vi "Инвертирование знака числа(5-разрядного).vi"(1 "A":T2) -> (0 "R":T1)   [LabVIEW 2013]
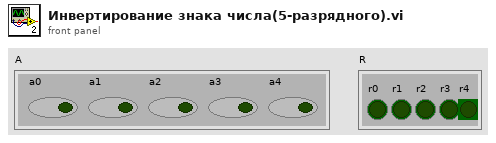
[diagram p1: front panel]
types:
  T1 = cluster{"r0":bool, "r1":bool, "r2":bool, "r3":bool, "r4":bool}
  T2 = cluster{"a0":bool, "a1":bool, "a2":bool, "a3":bool, "a4":bool}
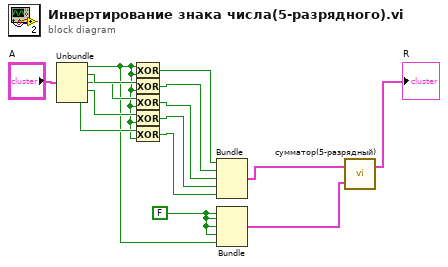
[diagram p0: block diagram]
diagram:
  w1 = FALSE
  n1 = Unbundle("A") -> ("a0"=w2:bool, "a1"=w14:bool, "a2"=w13:bool, "a3"=w12:bool, "a4"=w11:bool)
  n2 = Exclusive Or(1:w2, 2:w2) -> (0:w7:bool)
  n3 = Exclusive Or(1:w2, 2:w14) -> (0:w6:bool)
  n4 = Exclusive Or(1:w2, 2:w13) -> (0:w5:bool)
  n5 = Exclusive Or(1:w2, 2:w12) -> (0:w4:bool)
  n6 = Exclusive Or(1:w2, 2:w11) -> (0:w3:bool)
  n7 = Bundle(w7, w6, w5, w4, w3) -> (w10:cluster{bool, bool, bool, bool, bool})  [unwired: 1 in]
  n8 = Bundle(w1, w1, w1, w1, "a0"=w2) -> (w9:cluster{bool, bool, bool, bool, "a0":bool})  [unwired: 1 in]
  n9 = call "сумматор(5-разрядный).vi"("B"=w9, "A"=w10) -> ("R"=→"R":T1)  [unwired: 1 out]
